vi "Error Query.vi"(8 "error in (no error)":errorcluster, 11 "VISA resource name":refnum<visa-resource-name>) -> (0 "error out":errorcluster, 3 "VISA resource name out":refnum<visa-resource-name>)   [LabVIEW 2020, in "ScientiFic DC Power Supply.lvlib"]
doc: "Queries the instrument for any errors in the instrument's error queue. It will continue to read errors until all errors have been read from the instrument. Any errors will be returned in the <B>error out</B> control.\n\n<B>Note:</B>\nThis VI is called automatically by most driver VIs so it is not usually necessary to call this in an application."
uses:
  <instrlib>/ScientiFic DC Power Supply/ScientiFic DC Power Supply.lvlib
panel:
  # "EDIT: Note: The Error Query VI is included as a subVI in all driver VIs except low-level API VIs. If the instrument does not support error query, then remove the VI and remove subVI calls in each instrument driver VI that calls it."
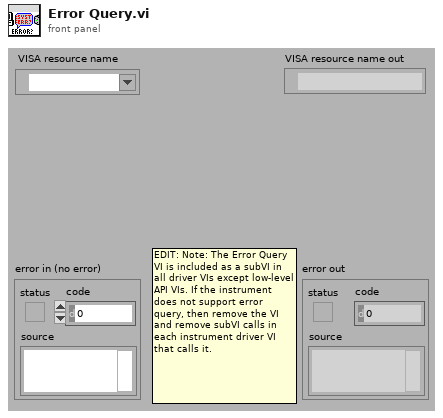
[diagram p1: front panel]
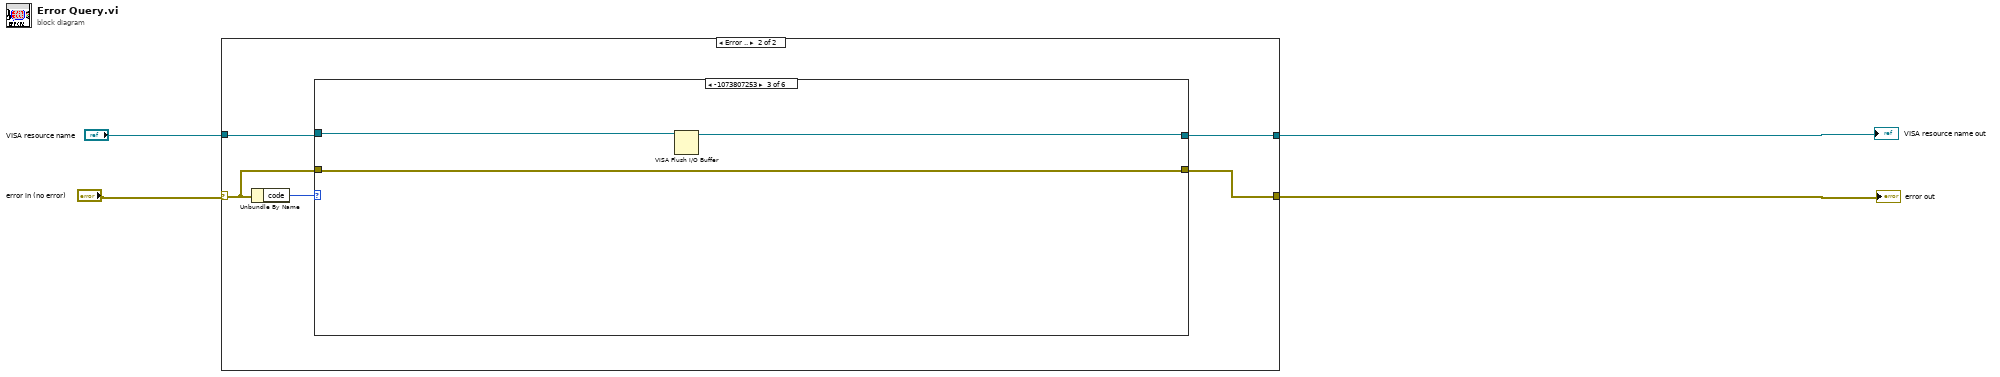
[diagram p0: block diagram]
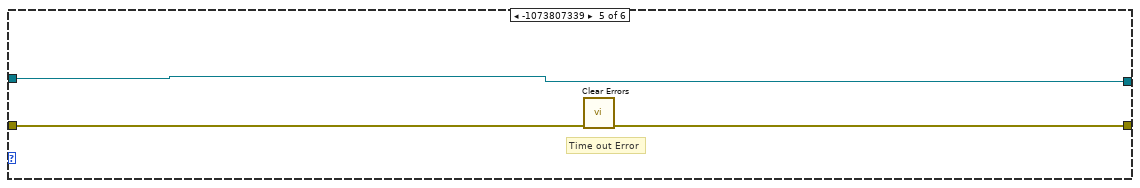
[diagram p6: hidden frame]
diagram:
  n1 = case shown="Error .." "error in (no error)" {
    selector: "error in (no error)" -> [w6 w10]
    tunnel: [w6 w9] -> w1
    tunnel: "VISA resource name" -> [w5 w8]
    tunnel: [w5 w7] -> w3
    frame No Error {
    }
    frame Error {
      n2 = Unbundle By Name(w10) -> ("code"=w11:i32)
      n3 = case shown="-1073807253" w11 {
        tunnel: w10 -> [w13 w14 w18 w20 w23 w24]
        tunnel: [w13 w14 w18 w20 w22 w24] -> w9
        tunnel: [w12 w15 w16 w19 w21 w25] -> w7
        tunnel: w8 -> [w12 w15 w17 w19 w21 w25]
        frame 0, Default {
        }
        frame -1073807194 {
        }
        frame -1073807253 {
          n4 = VISA Flush I/O Buffer(VISA resource name=w17) -> (VISA resource name out=w16:refnum<visa-resource-name>)  [unwired: 2 in, 1 out]
        }
        frame -1074004013 {
        }
        frame -1073807339 {
          # "Time out Error"
          n5 = call <vilib>:"Clear Errors.vi"("error in (no error)"=w23) -> ("error out"=w22:errorcluster)  [unwired: 5 in, 1 out]
        }
        frame -1073807343 {
        }
      }
    }
  }
  "VISA resource name out" <- w3
  "error out" <- w1
